vi "sbRIO.vi"() -> ()   [LabVIEW 2013]
uses:
  <vilib>/Platform/TimedLoop/XDataNode/timing_clust.ctl
  <vilib>/Platform/TimedLoop/XDataNode/nitl_modes.ctl
  <vilib>/Platform/TimedLoop/XDataNode/wakeup.ctl
  <vilib>/Analysis/coordinate.llb/Angle Units.ctl
  <vilib>/Analysis/coordinate.llb/Angle Range (Degree).ctl
  <vilib>/rvi/interface/common/niFpgaWaitOnOcc.vi
  <vilib>/Analysis/coordinate.llb/Wrap Angle (scalar).vi
  <vilib>/FPGAPlugInAG/sbRIO-9642/niLvFpga_Open_sbRIO-9642.vi
  <vilib>/rvi/interface/common/dynamic/niFpgaDynamicAddResources.vi
  <vilib>/Utility/error.llb/Error Cluster From Error Code.vi
  <vilib>/rvi/errors/niLvFpgaAdjustHostInterfaceError.vi
  <vilib>/FPGAPlugInAG/Dynamic/niLvFpga_Close_Dynamic.vi
  <vilib>/Platform/TimedLoop/XDataNode/XDataNode.xnode
  <vilib>/rvi/interface/nirviOpenFPGA/nirviOpenFPGA.xnode
  FPGA Bitfiles/ReleaseCandidate_FPGATarget_FPGA_LS4xwvBfOfc.lvbitx
  FPGA.vi
  <vilib>/rvi/interface/nirviReadWriteControl/nirviReadWriteControl.xnode
  <vilib>/rvi/interface/nirviCloseFPGA/nirviCloseFPGA.xnode
  NiFpgaLv.dll
  <vilib>/rvi/interface/Simulation/niFpgaSimulationCallBeginRW.vi
  Helper Functions/ProcessorHelperFunctions.lvlib
  <vilib>/Analysis/NI_AAL_Angle.lvlib
  <vilib>/Platform/TimedLoop/XDataNode/XDNodeRunTimeDep.lvlib
panel:
  in  "JoystickIn":i32[](array[numeric])
  in  "PID Gains":cluster{"P":dbl, "I":dbl, "D":dbl}={"P"=3.5, "I"=0.01, "D"=1.0}
  in  "Error Correction Speed":dbl=0.03
  out "Wheel Pos/Speed":picture
  out "Simulation Wheel Angles":dbl[](array[numeric])
  in  "Port":u16=2055 min=1025 step=1
  out "RX Data":T1
  in  "stop":bool
  in  "Manual Motor Control":bool=TRUE
  in  "Motor Number":u8
  out "Chassis Temp (C)":dbl
  out "E1":i64
  out "E3":i64
  out "E2":i64
  out "E4":i64
  out "A1":dbl
  out "A3":dbl
  out "A2":dbl
  out "A4":dbl
  out "T1":dbl
  out "T3":dbl
  out "T2":dbl
  out "T4":dbl
  in  "Calibration Mode":bool
  in  "Debug Mode":bool
  out "Wheel Target Angles":dbl[](array[numeric])
  out "Motor Output Values":u16[](array[slide]) scale=0.0..512.0
  in  "Offset1":i64=-77
  in  "Offset3":i64=108
  in  "Offset2":i64=-21
  in  "Offset4":i64=-108
  # "Manual Motor Control"
  # "Encoder Count Pre Offset"
  # "Override All"
  # "Automatic\n  Control"
  # "Actual Wheel Angles"
  # "Target Wheel Angles"
  # "Wheel Calibration offsets"
  # "Debug"
  # "(ECS models physical \nparamaters of the robot)"
  # "Normal Operation"
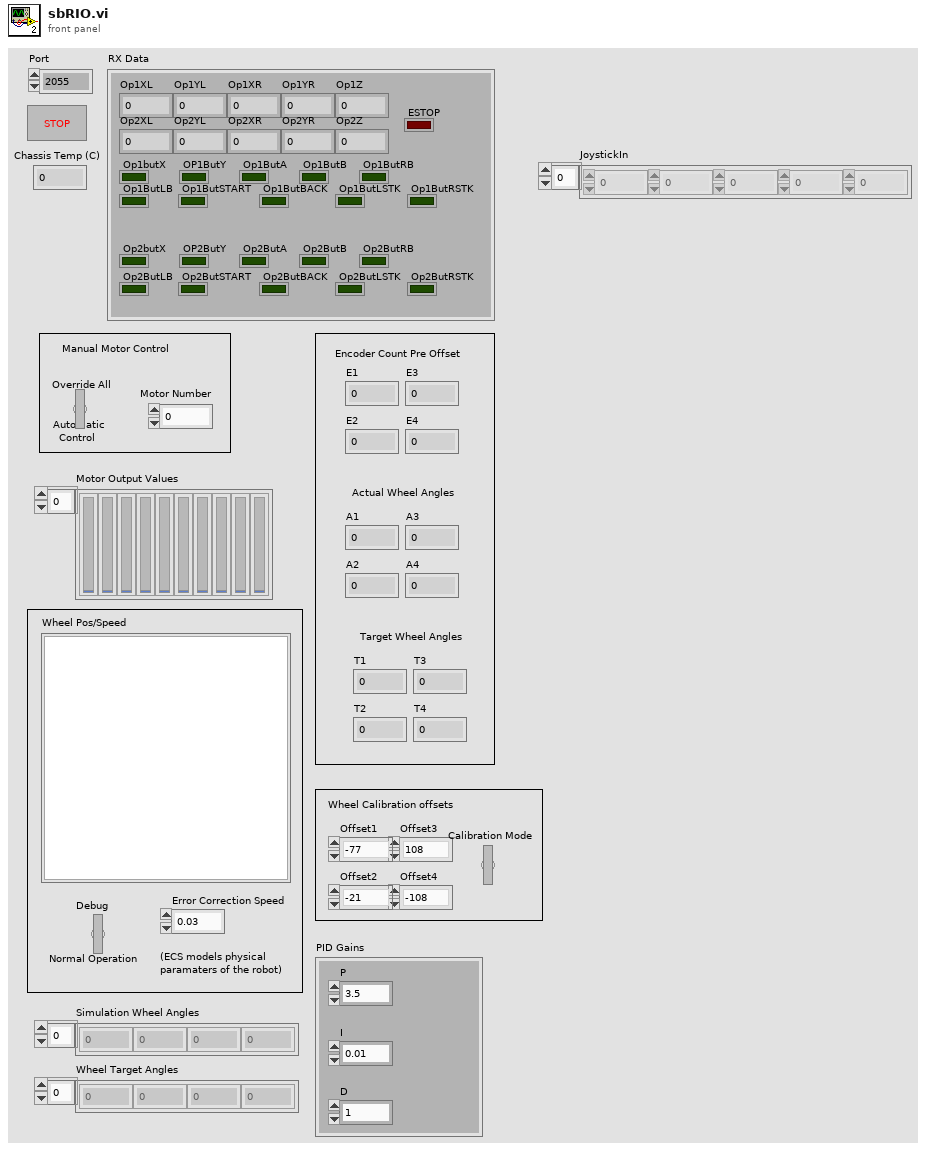
[diagram p1: front panel]
types:
  T1 = cluster{"Op2ButLSTK":bool, "Op2ButRSTK":bool, "Op1ButLSTK":bool, "Op1ButRSTK":bool, "Op1XL":i32, "Op1YL":i32, "Op1XR":i32, "Op1YR":i32, "Op1Z":i32, "Op2XL":i32, "Op2YL":i32, "Op2XR":i32, "Op2YR":i32, "Op2Z":i32, "ESTOP":bool, "Op1butX":bool, "OP1ButY":bool, "Op1ButA":bool, "Op1ButB":bool, "Op1ButRB":bool, "Op1ButLB":bool, "Op2butX":bool, "OP2ButY":bool, "Op2ButA":bool, "Op2ButB":bool, "Op2ButRB":bool, "Op2ButLB":bool, "Op2ButSTART":bool, "Op2ButBACK":bool, "Op1ButSTART":bool, "Op1ButBACK":bool}
  T2 = cluster{"MotorsOut[0]":u16, "MotorsOut[1]":u16, "MotorsOut[2]":u16, "MotorsOut[3]":u16}
  T3 = cluster{"Target Angles[0]":dbl, "Target Angles[1]":dbl, "Target Angles[2]":dbl, "Target Angles[3]":dbl}
  T4 = cluster{"MotorsOut[0]":u16, "MotorsOut[1]":u16, "MotorsOut[2]":u16, "MotorsOut[3]":u16, "MotorsOut[4]":u16, "MotorsOut[5]":u16, "MotorsOut[6]":u16, "MotorsOut[7]":u16, "MotorsOut[8]":u16, "MotorsOut[9]":u16, "MotorsOut[10]":u16, "MotorsOut[11]":u16}
  T5 = typedef "XDNodeRunTimeDep.lvlib/timing_clust.ctl" = cluster{"Expected End [f-1]":u64, "Actual End [f-1]":u64, "Finished Late? [f-1]":bool, "Expected End [i-1]":u64, "Actual End [i-1]":u64, "Finished Late? [i-1]":bool, "Expected Start [i]":u64, "Actual Start [i]":u64, "Expected Start [f]":u64, "Actual Start [f]":u64, "Source Name":string, "Structure Name":string, "Period":i64, "Deadline":i64, "Offset":i64, "Start":i64, "Priority":i32, "Timeout":i32, "Mode":T6, "Wakeup Reason":T7, "Error":errorcluster, "Source Type":string, "Secondary Source Type":string, "Global End Time":u64, "Global Start Time":u64, "Frame Duration":u64, "Iteration Duration":u64, "Assigned CPU":i32, "I/O Scan Engine Mode":u32}
  T6 = typedef "XDNodeRunTimeDep.lvlib/nitl_modes.ctl" = enum32{"No Change", "Process missed periods, maintain original phase", "Discard missed periods, maintain original phase", "Process missed periods, ignore original phase", "Discard missed periods, ignore original phase"}
  T7 = typedef "XDNodeRunTimeDep.lvlib/wakeup.ctl" = enum32{"Normal", "Aborted", "Asynchronous wakeup", "Timing source error", "Timed loop error", "Timeout"}
  T8 = typedef "NI_AAL_Angle.lvlib/Angle Range (Degree).ctl" = u16
  T9 = typedef "NI_AAL_Angle.lvlib/Angle Units.ctl" = i32
  T10 = cluster{"[0]":u16, "[1]":u16, "[2]":u16, "[3]":u16}
  T11 = cluster{"[0]":dbl, "[1]":dbl, "[2]":dbl, "[3]":dbl, "[4]":dbl, "[5]":dbl, "[6]":dbl, "[7]":dbl, "[8]":dbl}
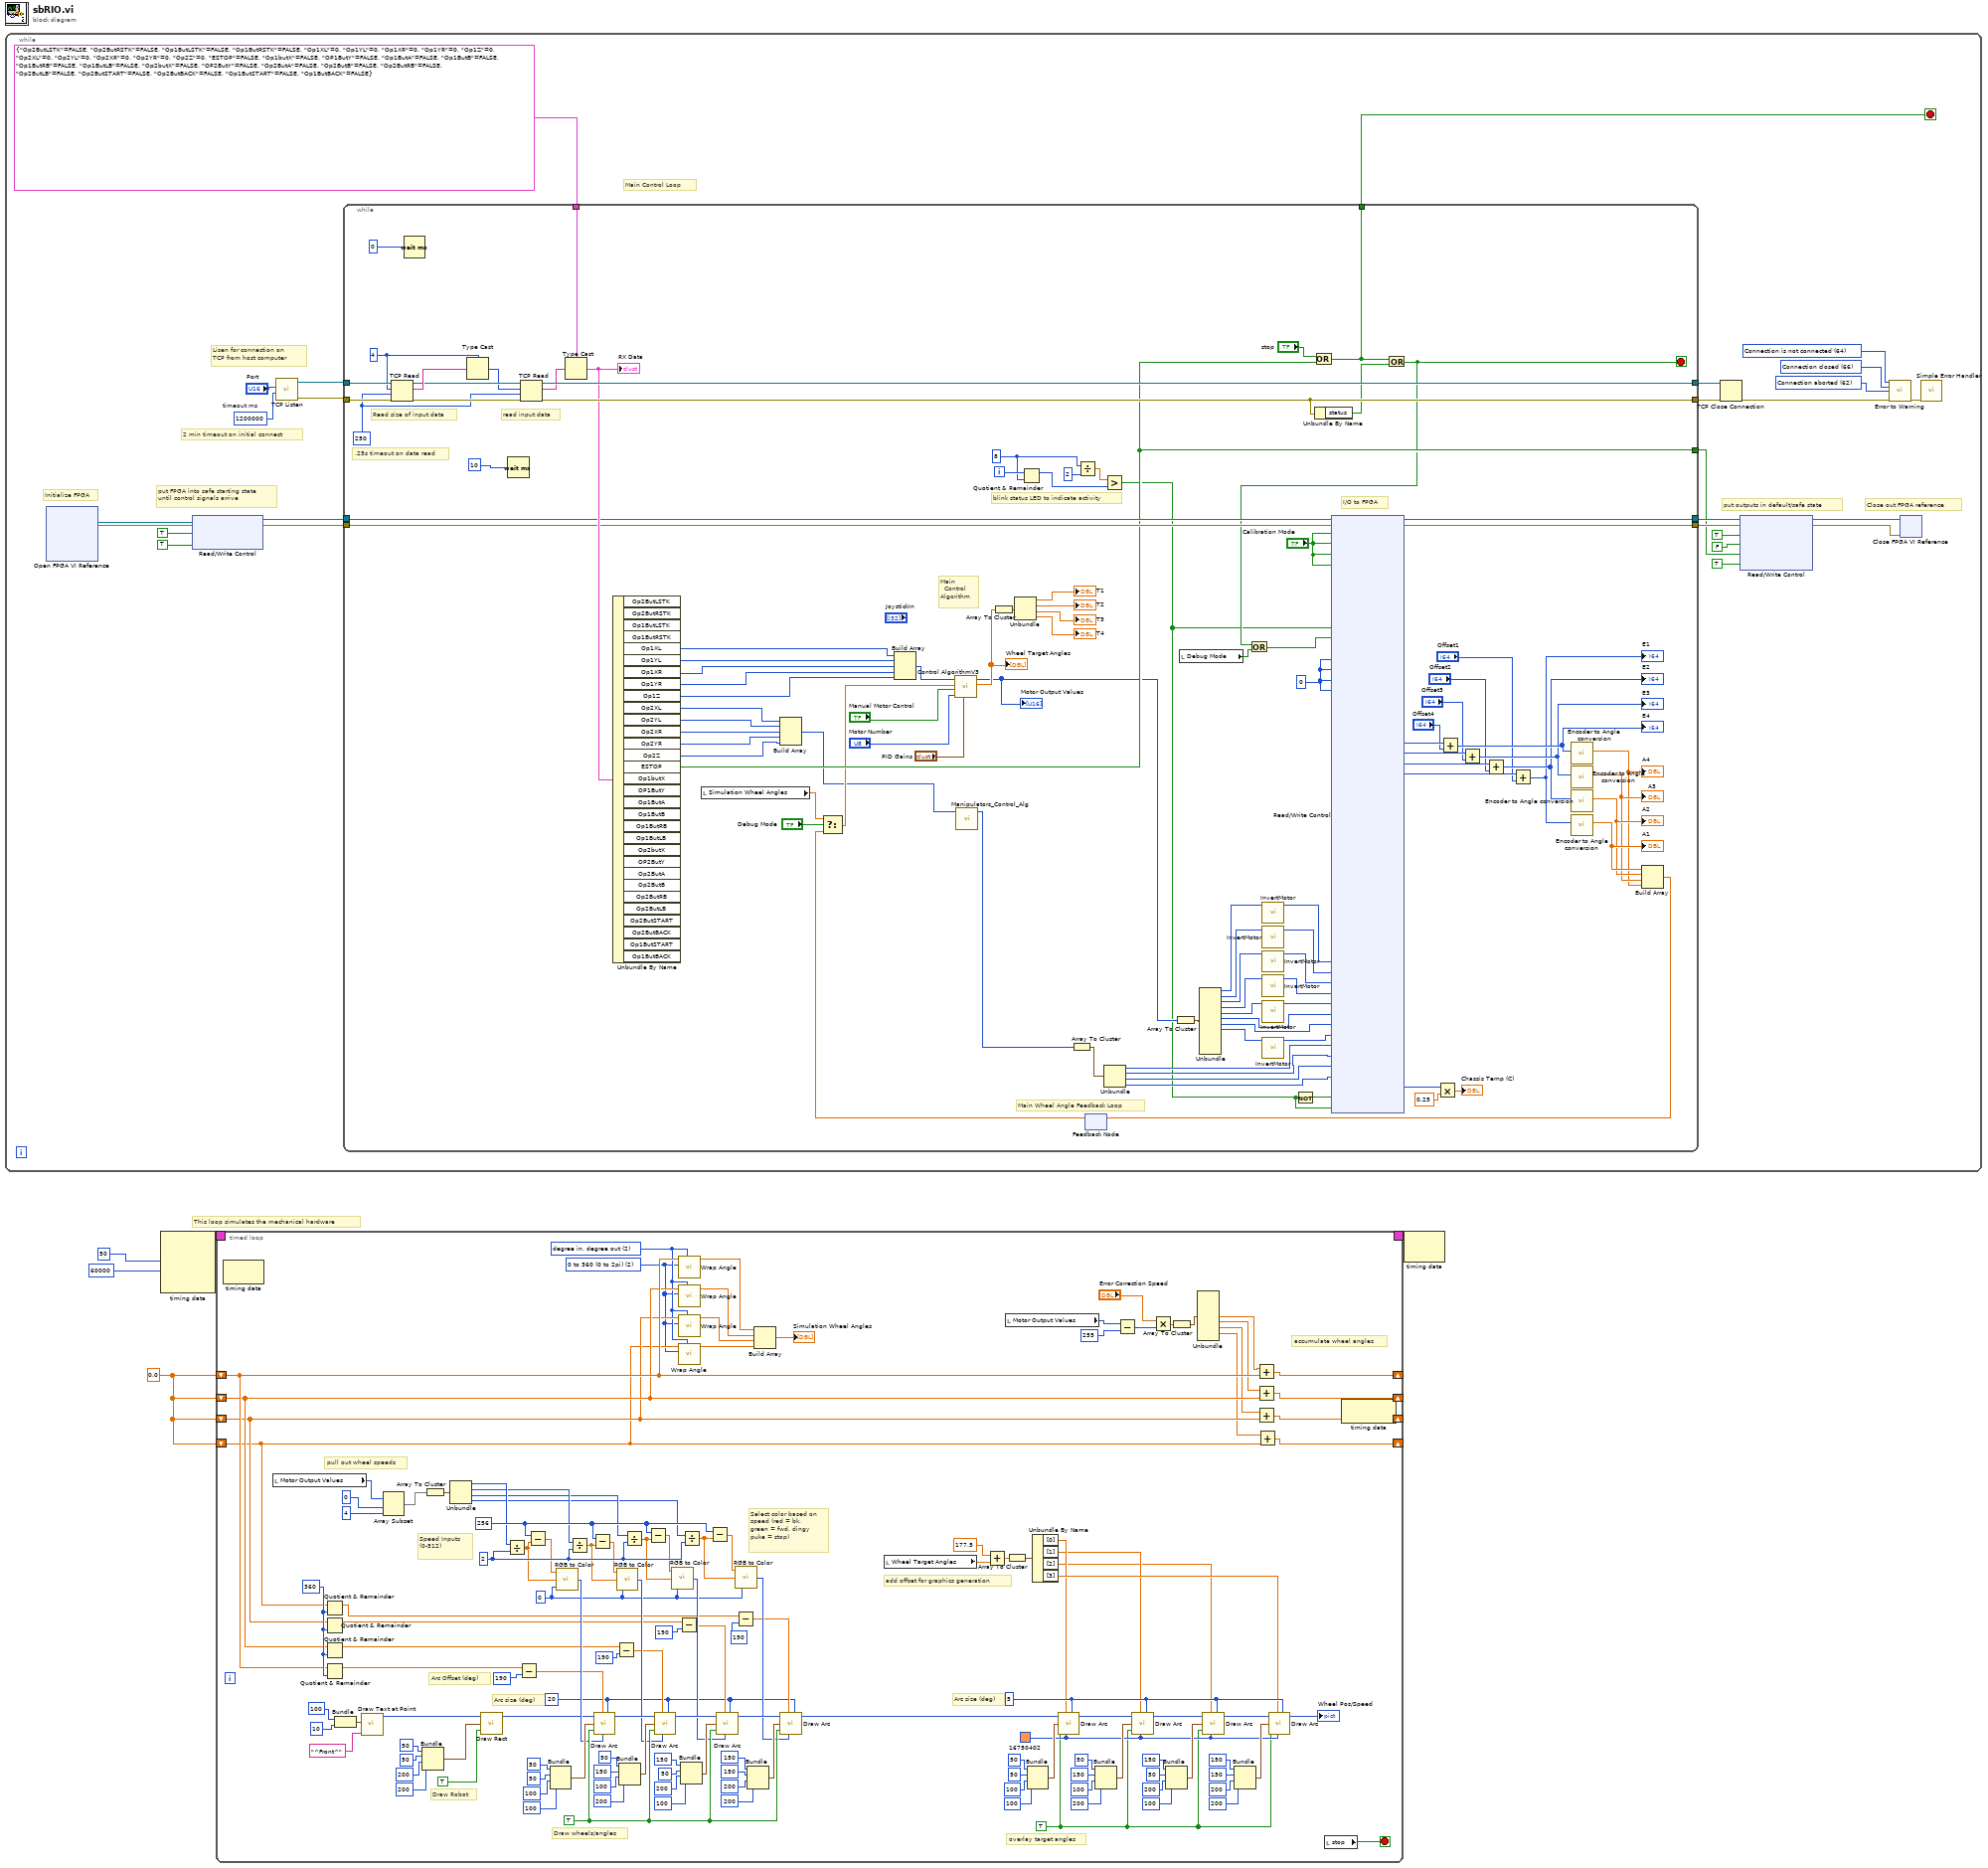
[diagram p0: block diagram]
diagram:
  w1 = 0.0
  # "This loop simulates the mechanical hardware"
  n1 = while {
    stop <- w6 stop-if-true
    w25 = 1200000  # timeout ms
    w29 = 62 items=["No Error", "Argument Error", "Memory Full", "Out of Zone", "End of File", "File Already Open", "Generic File IO Error", "File Not Found", "File Permission Error", "Disk Full", "Duplicate Path", "Too Many Files Open", "Not Enabled", "Resource File Not Found", "Cannot Add Resource", "Resource Not Found", "Image Not Found", "Image Memory Error", "Pen Does Not Exist", "Config Bad Type", "Config Token Not Found", "Config Parse Error", "Config Memory Error", "Bad External Code Format", "Bad External Code Offset", "External Code Not Present", "Null Window", "Destroy Window Mixup", "Null Menu", "Print Aborted", "Bad Print Record", "Print Driver Error", "Windows Error During Print", "Memory Error During Print", "Print Dialog Error", "Generic Print Error", "Invalid Device Refnum", "Device Not Found", "Device Parameter Error", "Device Unit Error", "Can't Open Device", "Device Call Aborted", "Generic Error", "Cancelled By User", "Object ID Too Low", "Object ID Too High", "Object Not In Heap", "Unknown Heap", "Bad DefProc ID", "DefProc Not In Table", "Message Out Of Range", "Null Method", "Unknown Message", "Manager Call Not Supported", "Bad address", "Connection In progress", "Connection timed out", "Connection is already in progress", "Network attribute not supported", "Network error", "Address in use", "System out of memory", "Connection aborted", "Connection refused", "Connection is not connected", "Connection is already connected", "Connection closed", "Initialize error (interapplication manager)", "Bad occurrence", "Wait on unbound occurrence handler", "Occurrence queue overflow", "Bad path", "Semaphore not signaled", "Unrecognized type (interapplication manager)"] ("1st Error to Convert")
    w30 = 66 items=["No Error", "Argument Error", "Memory Full", "Out of Zone", "End of File", "File Already Open", "Generic File IO Error", "File Not Found", "File Permission Error", "Disk Full", "Duplicate Path", "Too Many Files Open", "Not Enabled", "Resource File Not Found", "Cannot Add Resource", "Resource Not Found", "Image Not Found", "Image Memory Error", "Pen Does Not Exist", "Config Bad Type", "Config Token Not Found", "Config Parse Error", "Config Memory Error", "Bad External Code Format", "Bad External Code Offset", "External Code Not Present", "Null Window", "Destroy Window Mixup", "Null Menu", "Print Aborted", "Bad Print Record", "Print Driver Error", "Windows Error During Print", "Memory Error During Print", "Print Dialog Error", "Generic Print Error", "Invalid Device Refnum", "Device Not Found", "Device Parameter Error", "Device Unit Error", "Can't Open Device", "Device Call Aborted", "Generic Error", "Cancelled By User", "Object ID Too Low", "Object ID Too High", "Object Not In Heap", "Unknown Heap", "Bad DefProc ID", "DefProc Not In Table", "Message Out Of Range", "Null Method", "Unknown Message", "Manager Call Not Supported", "Bad address", "Connection In progress", "Connection timed out", "Connection is already in progress", "Network attribute not supported", "Network error", "Address in use", "System out of memory", "Connection aborted", "Connection refused", "Connection is not connected", "Connection is already connected", "Connection closed", "Initialize error (interapplication manager)", "Bad occurrence", "Wait on unbound occurrence handler", "Occurrence queue overflow", "Bad path", "Semaphore not signaled", "Unrecognized type (interapplication manager)"] ("1st Error to Convert")
    w31 = 64 items=["No Error", "Argument Error", "Memory Full", "Out of Zone", "End of File", "File Already Open", "Generic File IO Error", "File Not Found", "File Permission Error", "Disk Full", "Duplicate Path", "Too Many Files Open", "Not Enabled", "Resource File Not Found", "Cannot Add Resource", "Resource Not Found", "Image Not Found", "Image Memory Error", "Pen Does Not Exist", "Config Bad Type", "Config Token Not Found", "Config Parse Error", "Config Memory Error", "Bad External Code Format", "Bad External Code Offset", "External Code Not Present", "Null Window", "Destroy Window Mixup", "Null Menu", "Print Aborted", "Bad Print Record", "Print Driver Error", "Windows Error During Print", "Memory Error During Print", "Print Dialog Error", "Generic Print Error", "Invalid Device Refnum", "Device Not Found", "Device Parameter Error", "Device Unit Error", "Can't Open Device", "Device Call Aborted", "Generic Error", "Cancelled By User", "Object ID Too Low", "Object ID Too High", "Object Not In Heap", "Unknown Heap", "Bad DefProc ID", "DefProc Not In Table", "Message Out Of Range", "Null Method", "Unknown Message", "Manager Call Not Supported", "Bad address", "Connection In progress", "Connection timed out", "Connection is already in progress", "Network attribute not supported", "Network error", "Address in use", "System out of memory", "Connection aborted", "Connection refused", "Connection is not connected", "Connection is already connected", "Connection closed", "Initialize error (interapplication manager)", "Bad occurrence", "Wait on unbound occurrence handler", "Occurrence queue overflow", "Bad path", "Semaphore not signaled", "Unrecognized type (interapplication manager)"] ("1st Error to Convert")
    # "Main Control Loop"
    # "put FPGA into safe starting state\nuntil control signals arrive"
    # "put outputs in default/safe state"
    # "Close out FPGA reference"
    # "Initialize FPGA"
    # "2 min timeout on initial connect"
    # "Lisen for connection on \nTCP from host computer"
    n2 = xnode "Open FPGA VI Reference"() -> ("FPGA VI Reference Out"=w16:refnum<k20>, "error out"=w15:errorcluster)  [unwired: 2 in]
    n3 = xnode "Read/Write Control"("FPGA VI Reference In"=w16, "error in"=w15, "Stop All Motors"=TRUE, "Status LED"=TRUE) -> ("FPGA VI Reference Out"=w14:refnum<k20>, "error out"=w13:errorcluster)
    n4 = call <vilib>:"TCP Listen.vi"("timeout ms (wait forever: -1)"=w25, "port"="Port") -> ("error out"=w23:errorcluster, "connection ID"=w24:refnum<k5>)  [unwired: 5 in, 3 out]
    n5 = while {
      tunnel: w23 -> [w128]
      tunnel: w24 -> [w129]
      tunnel: [w130] -> w22
      tunnel: [w125] -> w21
      tunnel: T1 {"Op2ButLSTK"=FALSE, "Op2ButRSTK"=FALSE, "Op1ButLSTK"=FALSE, "Op1ButRSTK"=FALSE, "Op1XL"=0, "Op1YL"=0, "Op1XR"=0, "Op1YR"=0, "Op1Z"=0, "Op2XL"=0, "Op2YL"=0, "Op2XR"=0, "Op2YR"=0, "Op2Z"=0, "ESTOP"=FALSE, "Op1butX"=FALSE, "OP1ButY"=FALSE, "Op1ButA"=FALSE, "Op1ButB"=FALSE, "Op1ButRB"=FALSE, "Op1ButLB"=FALSE, "Op2butX"=FALSE, "OP2ButY"=FALSE, "Op2ButA"=FALSE, "Op2ButB"=FALSE, "Op2ButRB"=FALSE, "Op2ButLB"=FALSE, "Op2ButSTART"=FALSE, "Op2ButBACK"=FALSE, "Op1ButSTART"=FALSE, "Op1ButBACK"=FALSE} -> [w124]
      tunnel: w14 -> [w120]
      tunnel: w13 -> [w119]
      tunnel: [w118] -> w20
      tunnel: [w117] -> w19
      tunnel: [w111] -> w8
      tunnel: [w70] -> w6
      i -> [w116]
      stop <- w76 stop-if-true
      w93 = 0
      w112 = 8
      w123 = 250
      w126 = 4
      # "Main\n  Control\nAlgorithm"
      # "Main Wheel Angle Feedback Loop"
      # "blink status LED to indicate activity"
      # "I/O to FPGA"
      # ".25s timeout on data read"
      # "read input data"
      # "Read size of input data"
      n6 = TCP Read(connection ID=w129, bytes to read=w126, error in (no error)=w128, 9:w123) -> (connection ID out=w133:refnum<k5>, data out=w134:string, error out=w132:errorcluster)  [unwired: 1 in]
      n7 = Wait (ms)(milliseconds to wait=0) -> ()  [unwired: 1 out]
      n8 = Type Cast(type=w126, x=w134) -> (*(type *) &x=w131:i32)
      n9 = Wait (ms)(milliseconds to wait=10) -> ()  [unwired: 1 out]
      n10 = TCP Read(connection ID=w133, bytes to read=w131, error in (no error)=w132, 9:w123) -> (connection ID out=w130:refnum<k5>, data out=w127:string, error out=w125:errorcluster)  [unwired: 1 in]
      n11 = Type Cast(type=w124, x=w127) -> (*(type *) &x=w122:T1)
      "RX Data" <- w122
      n12 = Unbundle By Name(w122) -> ("Op1XL"=w81:i32, "Op1YL"=w80:i32, "Op1XR"=w79:i32, "Op1YR"=w78:i32, "Op1Z"=w77:i32, "Op2XL"=w46:i32, "Op2YL"=w45:i32, "Op2XR"=w44:i32, "Op2YR"=w43:i32, "Op2Z"=w42:i32, "ESTOP"=w111:bool)  [unwired: 20 out]
      n13 = local read "Simulation Wheel Angles"() -> (w90:dbl[])
      n14 = Build Array(w46, w45, w44, w43, w42) -> (w47:i32[])
      n15 = Build Array(w81, w80, w79, w78, w77) -> (w54:i32[])
      n16 = call "Manipulators_Control_Alg.vi"("Op2_Joysticks"=w47) -> ("MotorsOut"=w40:u16[])  [unwired: 10 in]
      n17 = Quotient & Remainder(x=w116, y=w112) -> (x-y*floor(x/y)=w114:i32)  [unwired: 1 out]
      n18 = Array To Cluster(array=w40) -> (cluster=w41:T2)
      n19 = Divide(x=w112, y=2) -> (x/y=w113:dbl)
      n20 = feedback #1() -> (w91:dbl[])  [unwired: 1 in]
      n21 = Select(t=w90, s="Debug Mode", f=w91) -> (s? t:f=w68:dbl[])
      n22 = call "Control AlgorithmV3.vi"("PID Gains"="PID Gains", "Motor to Control"="Motor Number", "Manual Control"="Manual Motor Control", "Wheel Angles"=w68, "JoystickIn"=w54) -> ("Target Angles"=w65:dbl[], "MotorsOut"=w64:u16[])  [unwired: 5 in]
      "Wheel Target Angles" <- w65
      "Motor Output Values" <- w64
      n23 = Array To Cluster(array=w65) -> (cluster=w106:T3)
      n24 = Unbundle(w106) -> ("Target Angles[0]"=→"T1":dbl, "Target Angles[1]"=→"T2":dbl, "Target Angles[2]"=→"T3":dbl, "Target Angles[3]"=→"T4":dbl)
      n25 = Greater?(x=w113, y=w114) -> (0:w35:bool)
      n26 = Unbundle(w41) -> ("MotorsOut[0]"=w39:u16, "MotorsOut[1]"=w38:u16, "MotorsOut[2]"=w37:u16, "MotorsOut[3]"=w36:u16)
      n27 = Array To Cluster(array=w64) -> (cluster=w110:T4)
      n28 = local read "Debug Mode"() -> (w74:bool)
      n29 = Unbundle(w110) -> ("MotorsOut[0]"=w62:u16, "MotorsOut[1]"=w56:u16, "MotorsOut[2]"=w58:u16, "MotorsOut[3]"=w60:u16, "MotorsOut[4]"=w52:u16, "MotorsOut[5]"=w51:u16, "MotorsOut[6]"=w48:u16, "MotorsOut[7]"=w50:u16)  [unwired: 4 out]
      n30 = call "InvertMotor.vi"("Input"=w62) -> ("Output"=w61:u16)  [unwired: 10 in]
      n31 = call "InvertMotor.vi"("Input"=w56) -> ("Output"=w55:u16)  [unwired: 10 in]
      n32 = call "InvertMotor.vi"("Input"=w58) -> ("Output"=w57:u16)  [unwired: 10 in]
      n33 = call "InvertMotor.vi"("Input"=w60) -> ("Output"=w59:u16)  [unwired: 10 in]
      n34 = call "InvertMotor.vi"("Input"=w52) -> ("Output"=w53:u16)  [unwired: 10 in]
      n35 = call "InvertMotor.vi"("Input"=w50) -> ("Output"=w49:u16)  [unwired: 10 in]
      n36 = Not(x=w35) -> (.not. x?=w73:bool)
      n37 = Or(x="stop", y=w111) -> (x .or. y?=w70:bool)
      n38 = Unbundle By Name(w125) -> ("status"=w69:bool)
      n39 = Or(x=w70, y=w69) -> (x .or. y?=w76:bool)
      n40 = Or(x=w76, y=w74) -> (x .or. y?=w75:bool)
      n41 = xnode "Read/Write Control"("FPGA VI Reference In"=w120, "error in"=w119, "Cal. 4"="Calibration Mode", "Cal. 3"="Calibration Mode", "Cal.2"="Calibration Mode", "Cal.1"="Calibration Mode", "Status LED"=w35, "Stop All Motors"=w75, "Analog 3"=w93, "Analog 1"=w93, "Analog 4"=w93, "Analog 2"=w93, "Motor1"=w61, "Motor2"=w55, "Motor3"=w57, "Motor4"=w59, "Motor5"=w53, "Motor6"=w51, "Motor7"=w48, "Motor8"=w49, "Motor9"=w39, "Motor10"=w38, "Motor11"=w37, "Motor12"=w36, "FPGA LED"=w73, "Watchdog_Kick"=w35) -> ("FPGA VI Reference Out"=w118:refnum<k20>, "error out"=w117:errorcluster, "Encoder4"=w72:i64, "Encoder3"=w101:i64, "Encoder2"=w100:i64, "Encoder1"=w99:i64, "Chasis Temp"=w107:i16)  [unwired: 14 in, 13 out]
      n42 = Multiply(x=w107, y=0.25) -> (x*y=→"Chassis Temp (C)":dbl)
      n43 = Add(x=w72, y="Offset4") -> (x+y=w88:i64)
      "E4" <- w88
      n44 = Add(x=w101, y="Offset3") -> (x+y=w87:i64)
      "E3" <- w87
      n45 = Add(x=w100, y="Offset2") -> (x+y=w86:i64)
      "E2" <- w86
      n46 = Add(x=w99, y="Offset1") -> (x+y=w85:i64)
      "E1" <- w85
      n47 = call "Encoder to Angle conversion.vi"("Input"=w88) -> ("Output"=w95:dbl)  [unwired: 10 in]
      "A4" <- w95
      n48 = call "Encoder to Angle conversion.vi"("Input"=w87) -> ("Output"=w96:dbl)  [unwired: 10 in]
      "A3" <- w96
      n49 = call "Encoder to Angle conversion.vi"("Input"=w86) -> ("Output"=w97:dbl)  [unwired: 10 in]
      "A2" <- w97
      n50 = call "Encoder to Angle conversion.vi"("Input"=w85) -> ("Output"=w98:dbl)  [unwired: 10 in]
      "A1" <- w98
      n51 = Build Array(w98, w97, w96, w95) -> (w94:dbl[])
      n52 = feedback-in #1(w94) -> ()
    }
    n53 = TCP Close Connection(connection ID=w22, error in (no error)=w21) -> (error out=w27:errorcluster)  [unwired: 1 in, 1 out]
    n54 = xnode "Read/Write Control"("FPGA VI Reference In"=w20, "error in"=w19, "Stop All Motors"=TRUE, "Status LED"=FALSE, "Emergency Stop"=w8, "Halt Execution"=TRUE) -> ("FPGA VI Reference Out"=w18:refnum<k20>, "error out"=w11:errorcluster)
    n55 = call <vilib>:"Error to Warning.vi"("1st Error to Convert"=w31, "2nd Error to Convert"=w30, "3rd Error to Convert"=w29, "error in"=w27) -> ("warning out"=w32:errorcluster)  [unwired: 11 in]
    n56 = xnode "Close FPGA VI Reference"("FPGA VI Reference In"=w18, "error in"=w11) -> ()  [unwired: 1 out]
    n57 = call <vilib>:"Simple Error Handler.vi"("error in (no error)"=w32) -> ()  [unwired: 4 in, 5 out]
  }
  n58 = node-c288(50, 60000) -> (w5:T5)  [unwired: 2 in]
  n59 = timed-loop {
    timing: w5 -> [_]
    timing-out: [_] -> w4
    shift-right: [w265] -> _
    shift-left: w1 -> [w147]
    shift-right: [w264] -> _
    shift-left: w1 -> [w146]
    shift-right: [w266] -> _
    shift-left: w1 -> [w148]
    shift-right: [w267] -> _
    shift-left: w1 -> [w149]
    stop <- w152 stop-if-true
    w139 = T8 2 items=["none", "-180 to 180 (-pi to pi)", "0 to 360 (0 to 2pi)"] ("angle range")
    w140 = T9 2 items=["radian in, radian out", "radian in, degree out", "degree in, degree out", "degree in, radian out"] ("angle units")
    w154 = 360
    w174 = TRUE
    w177 = 5
    w178 = u32 16750402
    w208 = 20
    w153 = 0
    w225 = 2
    w226 = 256
    w238 = TRUE
    # "add offset for graphics generation"
    # "pull out wheel speeds"
    # "Arc size (deg)"
    # "overlay target angles"
    # "Arc Offset (deg)"
    # "Arc size (deg)"
    # "Speed Inputs (0-512)"
    # "Draw wheels/angles"
    # "Select color based on speed (red = bk, green = fwd, dingy puke = stop)"
    # "Draw Robot"
    # "accumulate wheel angles"
    n60 = node-c288() -> ()  [unwired: 1 in, 1 out]
    n61 = local read "Motor Output Values"() -> (w165:u16[])
    n62 = Quotient & Remainder(x=w146, y=w154) -> (x-y*floor(x/y)=w158:dbl)  [unwired: 1 out]
    n63 = Quotient & Remainder(x=w147, y=w154) -> (x-y*floor(x/y)=w157:dbl)  [unwired: 1 out]
    n64 = Quotient & Remainder(x=w148, y=w154) -> (x-y*floor(x/y)=w156:dbl)  [unwired: 1 out]
    n65 = Quotient & Remainder(x=w149, y=w154) -> (x-y*floor(x/y)=w155:dbl)  [unwired: 1 out]
    n66 = Bundle(100, 10) -> (w203:cluster{i32, i32})  [unwired: 1 in]
    n67 = call <vilib>:"Draw Text at Point.vi"("text"="^Front^", "origin"=w203) -> ("new picture"=w207:picture)  [unwired: 8 in, 1 out]
    n68 = Array Subset(array=w165, index=0, length=4) -> (w170:u16[])
    n69 = Bundle(50, 50, 200, 200) -> (w229:cluster{i32, i32, i32, i32})  [unwired: 1 in]
    n70 = Array To Cluster(array=w170) -> (cluster=w171:T10)
    n71 = Unbundle(w171) -> ("[0]"=w169:u16, "[1]"=w168:u16, "[2]"=w167:u16, "[3]"=w166:u16)
    n72 = call <vilib>:"Draw Rect.vi"("picture"=w207, "rect"=w229, "fill?(F)"=TRUE) -> ("new picture"=w227:picture)  [unwired: 6 in]
    n73 = Divide(x=w169, y=w225) -> (x/y=w224:dbl)
    n74 = Subtract(x=w155, y=190) -> (x-y=w215:dbl)
    n75 = Subtract(x=w226, y=w224) -> (x-y=w221:dbl)
    n76 = Bundle(50, 50, 100, 100) -> (w255:cluster{i32, i32, i32, i32})  [unwired: 1 in]
    n77 = call <vilib>:"RGB to Color.vi"("B"=w153, "G"=w224, "R"=w221) -> ("Color"=w237:u32)
    n78 = Divide(x=w168, y=w225) -> (x/y=w223:dbl)
    n79 = Subtract(x=w226, y=w223) -> (x-y=w220:dbl)
    n80 = call <vilib>:"Draw Arc.vi"("picture"=w227, "start angle[degrees]"=w215, "rect"=w255, "fill?(F)"=w238, "color(black)"=w237, "arc size[degrees]"=w208) -> ("new picture"=w261:picture)  [unwired: 3 in]
    n81 = Subtract(x=w156, y=190) -> (x-y=w211:dbl)
    n82 = call <vilib>:"RGB to Color.vi"("B"=w153, "G"=w223, "R"=w220) -> ("Color"=w236:u32)
    n83 = Bundle(50, 150, 100, 200) -> (w241:cluster{i32, i32, i32, i32})  [unwired: 1 in]
    n84 = Divide(x=w167, y=w225) -> (x/y=w219:dbl)
    n85 = Subtract(x=w226, y=w219) -> (x-y=w218:dbl)
    n86 = call <vilib>:"Draw Arc.vi"("picture"=w261, "start angle[degrees]"=w211, "rect"=w241, "fill?(F)"=w238, "color(black)"=w236, "arc size[degrees]"=w208) -> ("new picture"=w260:picture)  [unwired: 3 in]
    n87 = call <vilib>:"RGB to Color.vi"("B"=w153, "G"=w219, "R"=w218) -> ("Color"=w235:u32)
    n88 = call-poly <vilib>:"Wrap Angle.vi"("angle units"=w140, "angle range"=w139, "angle in"=w149) -> ("angle out"=w145:dbl)  [unwired: 7 in, 1 out]
    n89 = call-poly <vilib>:"Wrap Angle.vi"("angle units"=w140, "angle range"=w139, "angle in"=w148) -> ("angle out"=w144:dbl)  [unwired: 7 in, 1 out]
    n90 = call-poly <vilib>:"Wrap Angle.vi"("angle units"=w140, "angle range"=w139, "angle in"=w147) -> ("angle out"=w143:dbl)  [unwired: 7 in, 1 out]
    n91 = call-poly <vilib>:"Wrap Angle.vi"("angle units"=w140, "angle range"=w139, "angle in"=w146) -> ("angle out"=w142:dbl)  [unwired: 7 in, 1 out]
    n92 = Subtract(x=w157, y=190) -> (x-y=w210:dbl)
    n93 = Bundle(150, 50, 200, 100) -> (w240:cluster{i32, i32, i32, i32})  [unwired: 1 in]
    n94 = Divide(x=w166, y=w225) -> (x/y=w222:dbl)
    n95 = Subtract(x=w226, y=w222) -> (x-y=w217:dbl)
    n96 = call <vilib>:"Draw Arc.vi"("picture"=w260, "start angle[degrees]"=w210, "rect"=w240, "fill?(F)"=w238, "color(black)"=w235, "arc size[degrees]"=w208) -> ("new picture"=w259:picture)  [unwired: 3 in]
    n97 = Subtract(x=w158, y=190) -> (x-y=w209:dbl)
    n98 = call <vilib>:"RGB to Color.vi"("B"=w153, "G"=w222, "R"=w217) -> ("Color"=w234:u32)
    n99 = Bundle(150, 150, 200, 200) -> (w239:cluster{i32, i32, i32, i32})  [unwired: 1 in]
    n100 = Build Array(w145, w144, w143, w142) -> (→"Simulation Wheel Angles":dbl[])
    n101 = call <vilib>:"Draw Arc.vi"("picture"=w259, "start angle[degrees]"=w209, "rect"=w239, "fill?(F)"=w238, "color(black)"=w234, "arc size[degrees]"=w208) -> ("new picture"=w202:picture)  [unwired: 3 in]
    n102 = local read "Wheel Target Angles"() -> (w164:dbl[])
    n103 = Add(x=177.5, y=w164) -> (x+y=w163:dbl[])
    n104 = local read "Motor Output Values"() -> (w150:u16[])
    n105 = Array To Cluster(array=w163) -> (cluster=w176:T11)
    n106 = Bundle(50, 50, 100, 100) -> (w196:cluster{i32, i32, i32, i32})  [unwired: 1 in]
    n107 = Unbundle By Name(w176) -> ("[0]"=w161:dbl, "[1]"=w160:dbl, "[2]"=w159:dbl, "[3]"=w175:dbl)
    n108 = call <vilib>:"Draw Arc.vi"("picture"=w202, "start angle[degrees]"=w161, "rect"=w196, "fill?(F)"=w174, "color(black)"=w178, "arc size[degrees]"=w177) -> ("new picture"=w201:picture)  [unwired: 3 in]
    n109 = Bundle(50, 150, 100, 200) -> (w190:cluster{i32, i32, i32, i32})  [unwired: 1 in]
    n110 = Subtract(x=w150, y=255) -> (x-y=w269:i32[])
    n111 = call <vilib>:"Draw Arc.vi"("picture"=w201, "start angle[degrees]"=w160, "rect"=w190, "fill?(F)"=w174, "color(black)"=w178, "arc size[degrees]"=w177) -> ("new picture"=w184:picture)  [unwired: 3 in]
    n112 = Multiply(x="Error Correction Speed", y=w269) -> (x*y=w263:dbl[])
    n113 = Bundle(150, 50, 200, 100) -> (w185:cluster{i32, i32, i32, i32})  [unwired: 1 in]
    n114 = Array To Cluster(array=w263) -> (cluster=w268:T11)
    n115 = Unbundle(w268) -> ("[4]"=w138:dbl, "[5]"=w137:dbl, "[6]"=w136:dbl, "[7]"=w135:dbl)  [unwired: 5 out]
    n116 = call <vilib>:"Draw Arc.vi"("picture"=w184, "start angle[degrees]"=w159, "rect"=w185, "fill?(F)"=w174, "color(black)"=w178, "arc size[degrees]"=w177) -> ("new picture"=w200:picture)  [unwired: 3 in]
    n117 = Bundle(150, 150, 200, 200) -> (w179:cluster{i32, i32, i32, i32})  [unwired: 1 in]
    n118 = Add(x=w138, y=w149) -> (x+y=w267:dbl)
    n119 = Add(x=w137, y=w148) -> (x+y=w266:dbl)
    n120 = Add(x=w136, y=w147) -> (x+y=w265:dbl)
    n121 = Add(x=w135, y=w146) -> (x+y=w264:dbl)
    n122 = call <vilib>:"Draw Arc.vi"("picture"=w200, "start angle[degrees]"=w175, "rect"=w179, "fill?(F)"=w174, "color(black)"=w178, "arc size[degrees]"=w177) -> ("new picture"=→"Wheel Pos/Speed":picture)  [unwired: 3 in]
    n123 = local read "stop"() -> (w152:bool)
    n124 = node-c288() -> ()  [unwired: 1 in, 1 out]
  }
  n125 = node-c288(w4) -> ()  [unwired: 1 out]
